vi "DigTemp - Read Temp.vi"(7 "Mode":enum16{"Config", "Temp?"}(ring), 8 "error in (no error)":errorcluster, 11 "PmodTMP3 address (x48)":u8=72 format="%x") -> (0 "error out":errorcluster, 2 "Bytes Read":u8[](array[numeric]), 3 "Temp":dbl)   [LabVIEW 2014]
uses:
  <vilib>/myRIO/Instrument Drivers/Onboard IO/I2C/vis/Configure.vi
  <vilib>/myRIO/Instrument Drivers/Onboard IO/I2C/vis/Write Read.vi
  <vilib>/myRIO/Instrument Drivers/Onboard IO/I2C/vis/Read.vi
  <vilib>/myRIO/Instrument Drivers/Onboard IO/I2C/vis/Smart Open.vi
  <vilib>/Utility/error.llb/Error Cluster From Error Code.vi
  <vilib>/myRIO/Common/Instrument Driver Framework/myRIO v1.0/I2C/vis/myRIO v1.0 Configure I2C.vi
  <vilib>/myRIO/Common/Instrument Driver Framework/myRIO v1.0/I2C/vis/myRIO v1.0 Write I2C.vi
  <vilib>/myRIO/Common/Instrument Driver Framework/myRIO v1.0/I2C/vis/myRIO v1.0 Read I2C.vi
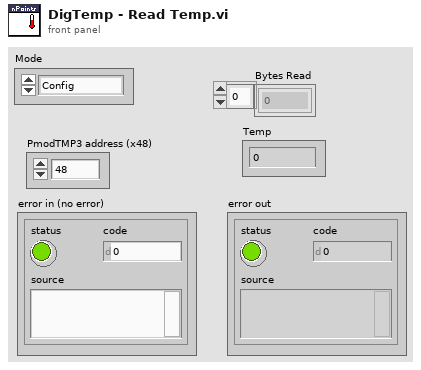
[diagram p1: front panel]
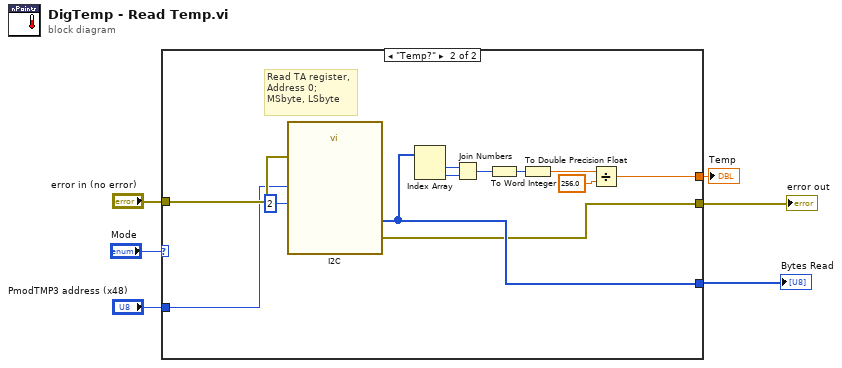
[diagram p0: block diagram]
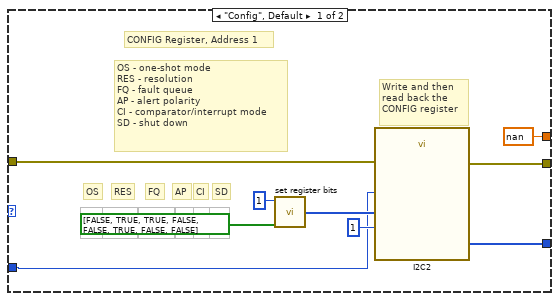
[diagram p2: hidden frame]
diagram:
  n1 = case shown="\"Temp?\"" "Mode" {
    tunnel: "error in (no error)" -> [w10 w24]
    tunnel: [nan w23] -> w5
    tunnel: "PmodTMP3 address (x48)" -> [w11 w18]
    tunnel: [w7 w17] -> w2
    tunnel: [w9 w16] -> w1
    frame "Config", Default {
      # "Write and then\nread back the\nCONFIG register"
      # "OS - one-shot mode\nRES - resolution\nFQ - fault queue\nAP - alert polarity\nCI - comparator/interrupt mode\nSD - shut down"
      # "SD"
      # "CI"
      # "AP"
      # "FQ"
      # "RES"
      # "OS"
      # "CONFIG Register, Address 1"
      n2 = call "set register bits.vi"("address"=u8 1, "register bits"=bool[] [FALSE, TRUE, TRUE, FALSE, FALSE, TRUE, FALSE, FALSE]) -> ("address / value"=w14:u8[])  [unwired: 5 in]
      n3 = call "I2C2"("Slave Address (7-bit)"=w11, "Bytes to Write"=w14, "Byte Count"=u32 1, "error in (no error)"=w10) -> ("Bytes Read"=w7:u8[], "error out"=w9:errorcluster)  [unwired: 22 in]
    }
    frame "Temp?" {
      # "Read TA register,\nAddress 0;\nMSbyte, LSbyte"
      n4 = call "I2C"("Slave Address (7-bit)"=w18, "Byte Count"=u32 2, "error in (no error)"=w24) -> ("Bytes Read"=w17:u8[], "error out"=w16:errorcluster)  [unwired: 23 in]
      n5 = Index Array(array=w17) -> (element #1=w21:u8, element #2=w22:u8)  [unwired: 2 in]
      n6 = Join Numbers(hi=w21, lo=w22) -> ((hi.lo)=w25:u16)
      n7 = To Word Integer(number=w25) -> (16bit integer=w26:i16)
      n8 = To Double Precision Float(number=w26) -> (double precision float=w19:dbl)
      n9 = Divide(x=w19, y=256.0) -> (x/y=w23:dbl)
    }
  }
  "Temp" <- w5
  "Bytes Read" <- w2
  "error out" <- w1
